vi "TurtleModeSailSuggestion.vi"(9 "AbsoluteWindAngle":dbl, 10 "BoatVelocity":dbl, 11 "RelativeWindAngle":dbl) -> (2 "Suggested Rudder Setpoint":T2 min=-1.0 max=1.0, 3 "Suggested Sail Setpoints":T1 {"MainSailSuggestion" min=0.0 max=1.0; "JibSailSuggestion" min=0.0 max=1.0})   [LabVIEW 2012]
doc: "Suggests sail and rudder settings that will keep the boat safe in high winds.\n\nThis should most likely be done by trying to keep the sails perpendicular to the wind and maybe using the rudder to turn the boat into the wind when possible. Locking the rudder in place is also a possibility."
uses:
  Data/TypeDefs/Sail Set Suggestions.ctl
  Data/TypeDefs/Rudder Set Suggestions.ctl
panel:
  # "Suggests sail and rudder settings that\nwill keep the boat safe in high winds.\n\nTODO: his should most likely be done by trying\nto keep the sails perpendicular to the wind\nand maybe using the rudder to turn the\nboat into the wind when possible. Locking\nthe rudder in place is also a possibility.\n\nThe decision for whether to go into turtle mode\nis NOT made here, that is done in\nDetermineStateOfBoat.vi"
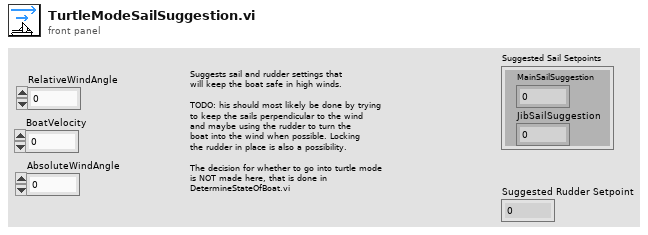
[diagram p1: front panel]
types:
  T1 = typedef "Sail Set Suggestions.ctl" = cluster{"MainSailSuggestion":dbl, "JibSailSuggestion":dbl}
  T2 = typedef "Rudder Set Suggestions.ctl" = dbl
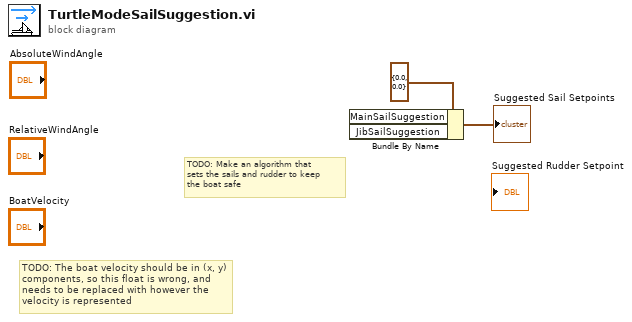
[diagram p0: block diagram]
diagram:
  # "TODO: Make an algorithm that\nsets the sails and rudder to keep\nthe boat safe"
  # "TODO: The boat velocity should be in (x, y)\ncomponents, so this float is wrong, and\nneeds to be replaced with however the\nvelocity is represented"
  n1 = Bundle By Name(cluster=T1 {"MainSailSuggestion"=0.0, "JibSailSuggestion"=0.0} ("output cluster")) -> (→"Suggested Sail Setpoints":T1)  [unwired: 2 in]
